vi "max-search.vi"() -> ()   [LabVIEW 2025]
panel:
  out "Max":dbl
  out "Iterations":i32
  in  "Number of Iterations":i32
  out "Random Number":dbl
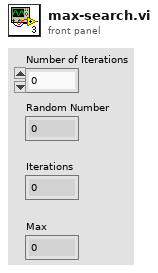
[diagram p1: front panel]
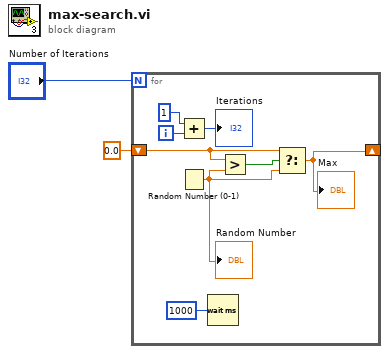
[diagram p0: block diagram]
diagram:
  n1 = for {
    N: "Number of Iterations" -> [_]
    shift-right: [w3] -> _
    shift-left: 0.0 -> [w5]
    i -> [w9]
    n2 = Add(x=1, y=w9) -> (x+y=→"Iterations":i32)
    n3 = Random Number (0-1)() -> (number: 0 to 1=w4:dbl)
    "Random Number" <- w4
    n4 = Wait (ms)(milliseconds to wait=u32 1000) -> ()  [unwired: 1 out]
    n5 = Greater?(x=w5, y=w4) -> (0:w6:bool)
    n6 = Select(t=w5, s=w6, f=w4) -> (s? t:f=w3:dbl)
    "Max" <- w3
  }
